vi "Set_Action.vi"(8 "error in (no error)":errorcluster caption="entrée d'erreur (pas d'erreur)", 10 "Action":T1, 11 "Class Instrument Power_Supply en entrée":refnum<class "Class Instrument Power_Supply.lvclass">) -> (0 "error out":errorcluster caption="sortie d'erreur", 3 "Class Instrument Power_Supply en sortie":refnum<class "Class Instrument Power_Supply.lvclass">)   [LabVIEW 2020, in "Library Instrument & Equipement.lvlib" / "Library Instruments.lvlib" / "Class Instrument Power_Supply.lvclass"]
uses:
  Class Instrument Power_Supply.lvclass
  Commun VI/TypeDef/Command Power_Supply/Data_Write_Power_Supply.ctl
  Class Instrument Power_Supply.lvclass/Class Instrument Power_Supply.ctl
  Commun VI/Library Commun.lvlib
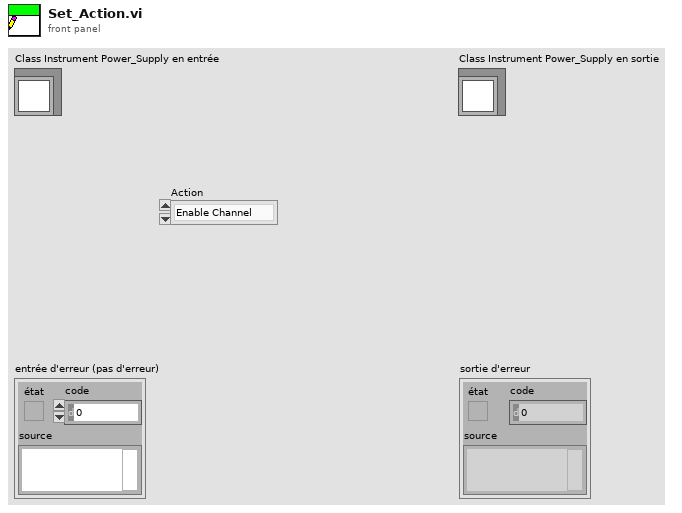
[diagram p1: front panel]
types:
  T1 = typedef "Library Commun.lvlib/Data_Write_Power_Supply.ctl" = enum16{"Enable Channel", "Disable Channel"}
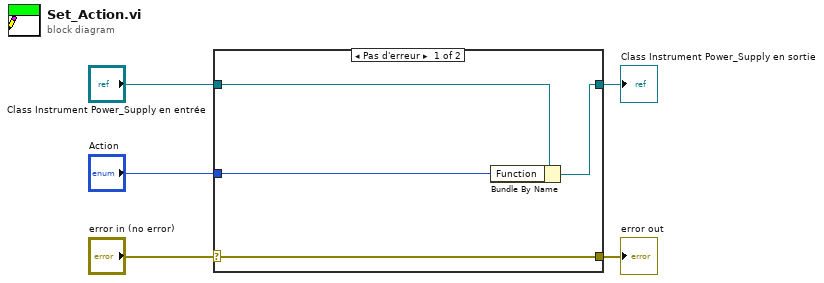
[diagram p0: block diagram]
diagram:
  n1 = case shown="Pas d'erreur" "error in (no error)" {
    selector: "error in (no error)" -> [w9 w10]
    tunnel: [w9 w10] -> w4
    tunnel: [w7 w11] -> w2
    tunnel: "Class Instrument Power_Supply en entrée" -> [w8 w11]
    tunnel: "Action" -> [w6 _]
    frame No Error {
      n2 = Bundle By Name(cluster=w8, "Function"=w6) -> (w7:refnum<class "Class Instrument Power_Supply.lvclass">)
    }
    frame Error {
    }
  }
  "error out" <- w4
  "Class Instrument Power_Supply en sortie" <- w2
